vi "Convert to PSI.vi"(11 "Raw V":dbl) -> (3 "Pressure(psi)":dbl)   [LabVIEW 2020]
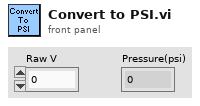
[diagram p1: front panel]
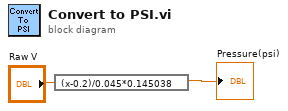
[diagram p0: block diagram]
diagram:
  n1 = expression code="(x-0.2)/0.045*0.145038"("Raw V") -> (→"Pressure(psi)":dbl)
